vi "Configure.vi"(6 "High Level Config Settings in":T2={"Default Refresh Rate (ms)"=500, "Show Border"=FALSE, "Periodic Decoration Data"=FALSE, "Synchronous Requests"=FALSE, "Reduce Sent Data"=FALSE, "Recommended Control Settings"=FALSE}, 7 "Default Control Behavior":T3, 8 "error in (no error)":errorcluster, 10 "Config Option":T4, 11 "reference in":refnum<class "Web Front Panel.lvclass">) -> (0 "error out":errorcluster, 3 "reference out":refnum<class "Web Front Panel.lvclass">)   [LabVIEW 2017, in "Front Panel Publisher.lvlib" / "Web Front Panel.lvclass"]
doc: "Configure the options for the web-representation of the front panel"
uses:
  Web Front Panel.lvclass
  Controls/FP Object Configuration.ctl
  Common/Enum - Config Option.ctl
  Controls/Cluster - Default Control Behavior.ctl
  Controls/High Level Config Settings.ctl
  Web Front Panel.lvclass/Web Front Panel.ctl
  <vilib>/Utility/error.llb/DialogType.ctl
  Front Panel Objects/Object_class/Object.lvclass
  Front Panel Publisher.lvlib
panel:
  in  "Control Instructions":T1(tab)
  in  "Exit":bool
  in  "Save":bool
  in  "Tab Control":enum32{"Base Config", "Controls", "Indicators"}(tab)
  in  "High Level Config Settings":T2={"Default Refresh Rate (ms)"=750, "Show Border"=FALSE, "Periodic Decoration Data"=FALSE, "Synchronous Requests"=FALSE, "Reduce Sent Data"=FALSE, "Recommended Control Settings"=FALSE}
  in  "Controls":T5[](array[typedef])
  in  "Indicators":T5[](array[typedef])
  # "All controls and indicators can be represented as an image.  Sending a control state as an image means it cannot be interacted with in the web page, and large amounts of data are sent since the whole image is sent instead of just the control value.  This is the Control is Image setting.  This will send just the image but no position or visibility.\n\nThe Image and Visibility will send both the control image, and the position and visibility with each request.  This means if a control is hidden, moved, or resized while the VI is running, the new attributes will be sent automatically.\n\nIf a control is set to Control is Image the position, size, and visibility can be forced to be sent using the Force Update VI.\n\nSince booleans only have two image states, they cannot have the image modes and instead have special Boolean Modes."
  # "When a control is set to Value Only the control's changed position, size or other attributes will not be sent, just the value.  These values will be represented as native web controls and will have the look of the web equivalent control.\n\nThe value is read using get Control Value By Index when possible, but ideally uses no properties or methods on the control.\n\nIf a control is set to Value and Visibility, then value position, size, and other attributes wil be sent with each request.\n\nIf a control is set to Value Only the position, size, and other attributes can be forced to be sent using the Force Update VI."
  # "A Boolean can be set to Value Only, or Value and Visibility like some other controls.  This will have the boolean seen with the web button equivalent.  However since a boolean only has two states there is also the Boolean Value Only which operates like Value Only, except that the two boolean states are seen as images in the webpage, but only send a True or False and not the whole image with each request.\n\nBooleans also have another mode called Boolean Value and Visibility which mirrors the Value and Visibility in that it sends the value, position, size, and other attributes with each request.\n\nIf a control is set to Boolean Value Only the position, size, and other attributes can be forced to be sent using the Force Update VI."
  # "Default Refresh Rate - This is the rate that the page will request new data.  This can be change by clicking the cog in the lower right corner.\n\nShow Border - This will make a border the size of the FP window.\n\nPeriodic Decoration Data - If enabled, then with every request, all decoration positions, size, visibility, and text will be sent and updated.  If false this information will only be updated if a Force Update is used.  Free text is considered a decoration.\n\nSynchronous Requests - This ensures that a request for data won't be sent unless the previous request has been returned.  This is useful at times, but if a reply is lost for some reason the page will hang.\n\nReduce Sent Data - This will reduce the amount of data sent, by only sending data that has changed since the last request from each connection.  This does reduce the amount of data sent, but also increases the time it takes to send a reply."
  # "Control Label"
  # "Control Type"
  # "Display Mode"
  # "Control Label"
  # "Control Type"
  # "Display Mode"
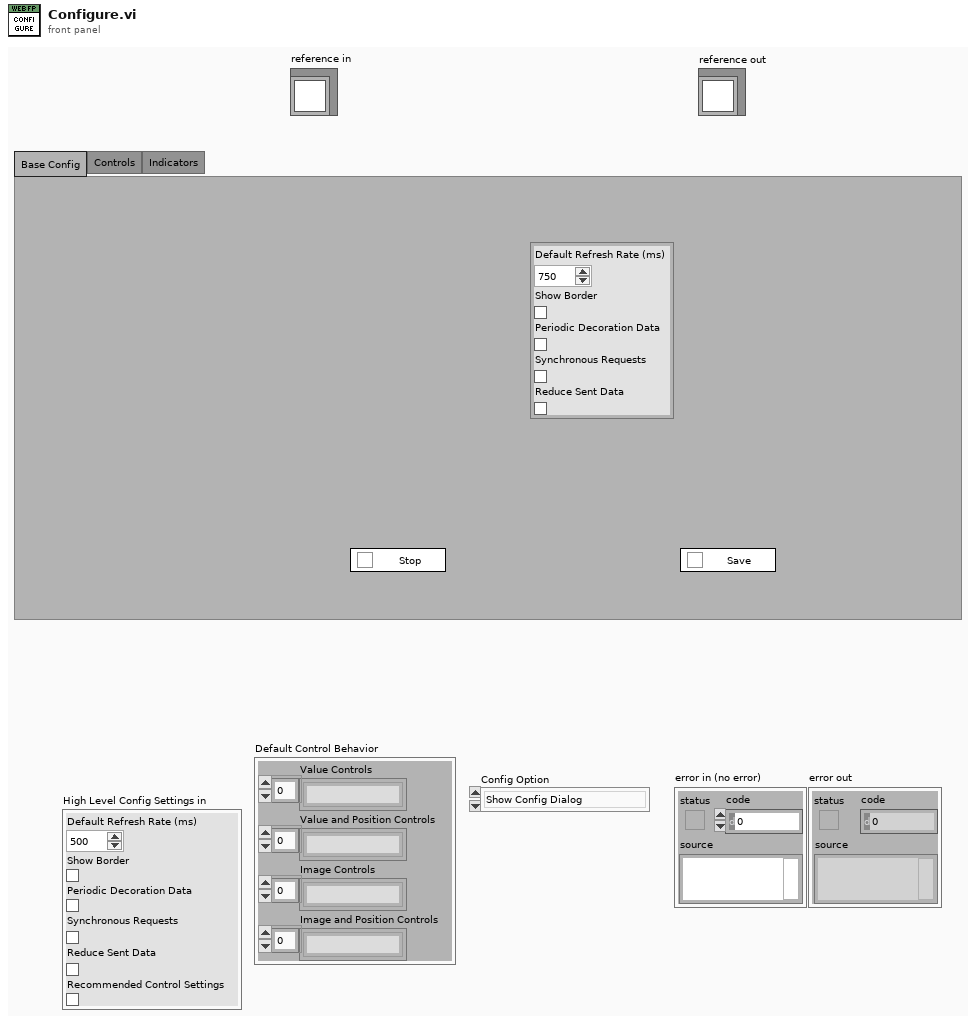
[diagram p1: front panel]
types:
  T1 = enum32{"Image Modes", "Value Modes", "Boolean Modes"}
  T2 = typedef "Front Panel Publisher.lvlib/Web Front Panel.lvclass/High Level Config Settings.ctl" = cluster{"Default Refresh Rate (ms)":i32, "Show Border":bool, "Periodic Decoration Data":bool, "Synchronous Requests":bool, "Reduce Sent Data":bool, "Recommended Control Settings":bool}
  T3 = typedef "Front Panel Publisher.lvlib/Web Front Panel.lvclass/Cluster - Default Control Behavior.ctl" = cluster{"Value Controls":string[], "Value and Position Controls":string[], "Image Controls":string[], "Image and Position Controls":string[]}
  T4 = typedef "Front Panel Publisher.lvlib/Enum - Config Option.ctl" = enum16{"Show Config Dialog", "Don't Show Config Dialog", "Load Config File then Show Dialog", "Load Config File No Dialog"}
  T5 = typedef "Front Panel Publisher.lvlib/Web Front Panel.lvclass/FP Object Configuration.ctl" = cluster{"Name":string, "Control Type":string, "Display Mode":string}
  T6 = enum32{"Invalid", "Standard", "Closed", "Hidden", "Minimized", "Maximized"}
  T7 = typedef "LVPoint32TypeDef.ctl" = cluster{"Horizontal":i32, "Vertical":i32}
  T8 = typedef "Front Panel Publisher.lvlib/Web Front Panel.lvclass/Object Attributes.ctl" = cluster{"VI Identifier":string, "VI Reference":refnum<vi>, "Controls":refnum<class "Object.lvclass">[], "Indicators":refnum<class "Object.lvclass">[], "Decorations":refnum<class "Object.lvclass">[], "VR With Previous Get":refnum<data-value>, "VR With Ring Images":refnum<data-value>}
  T9 = typedef "DialogType.ctl" = u16
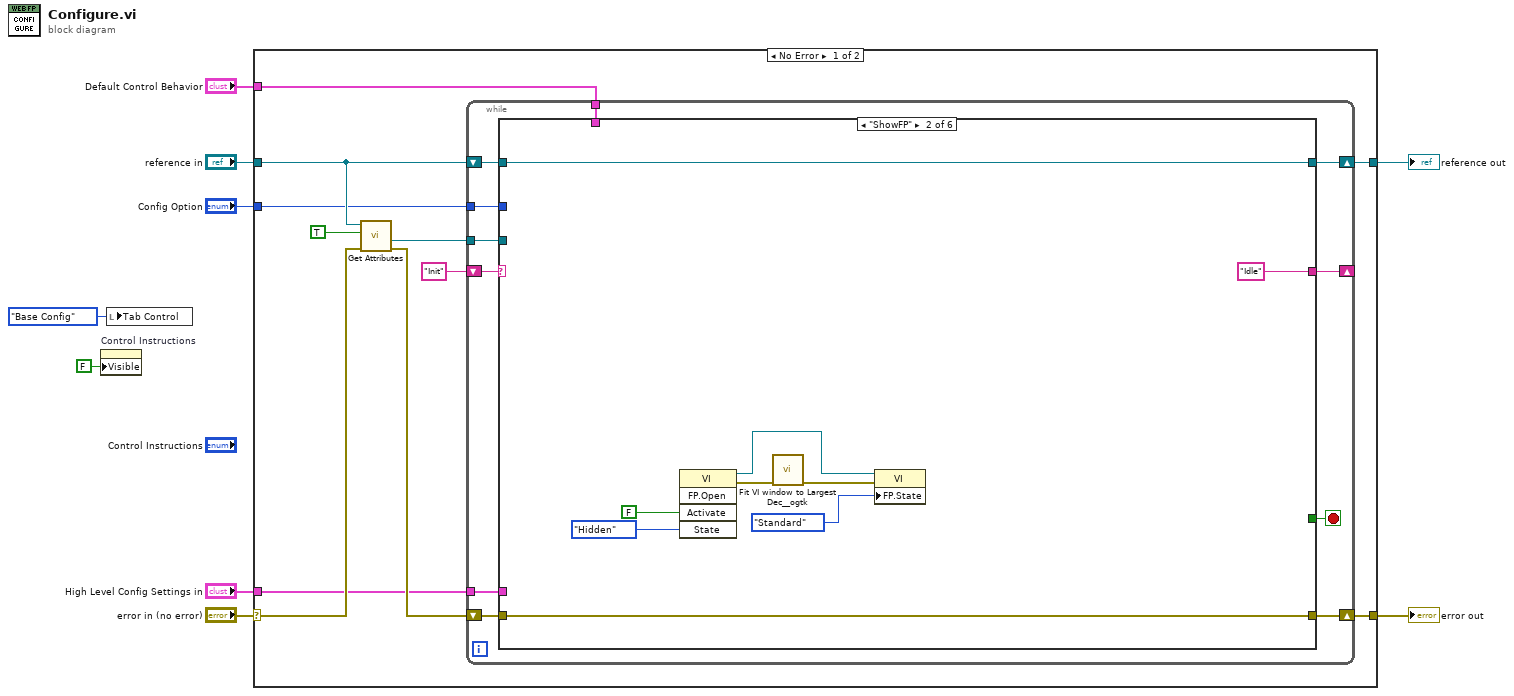
[diagram p0: block diagram]
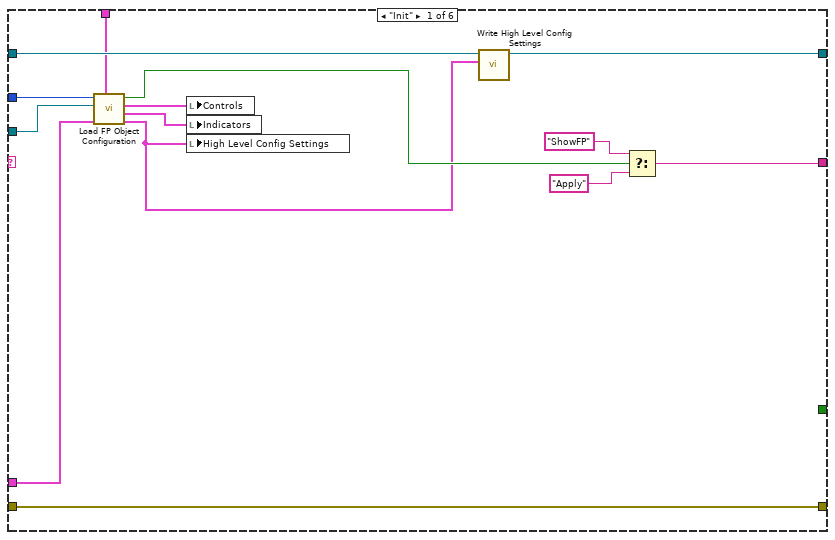
[diagram p2: hidden frame]
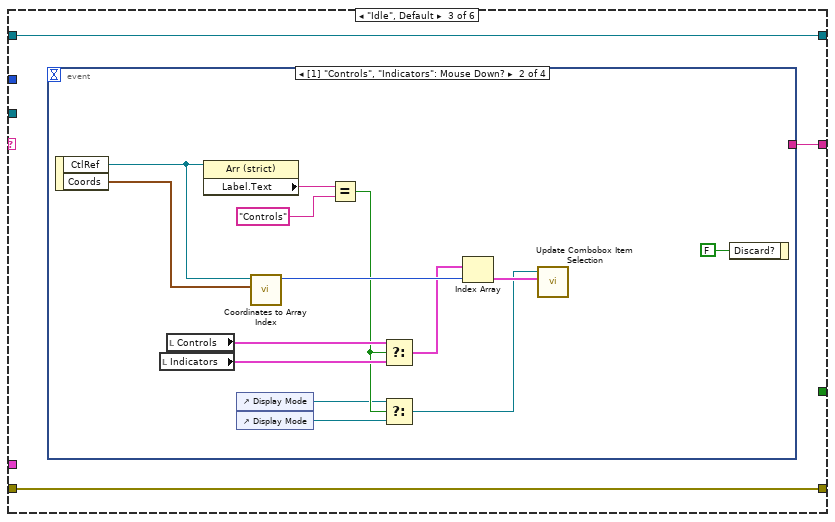
[diagram p3: hidden frame]
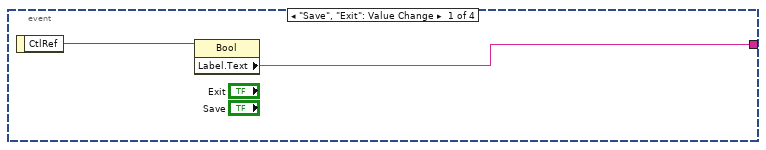
[diagram p4: hidden frame]
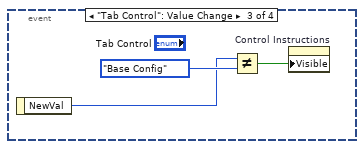
[diagram p5: hidden frame]
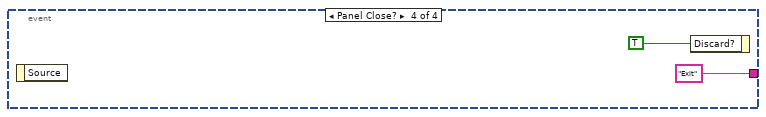
[diagram p6: hidden frame]
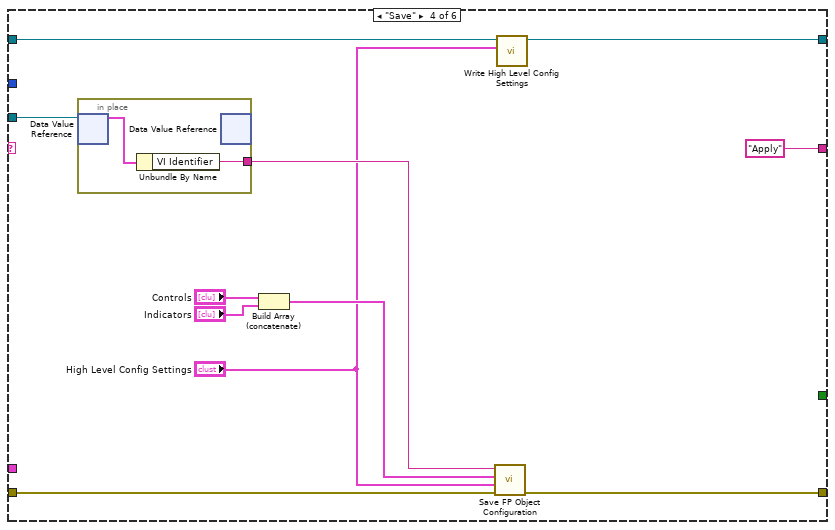
[diagram p7: hidden frame]
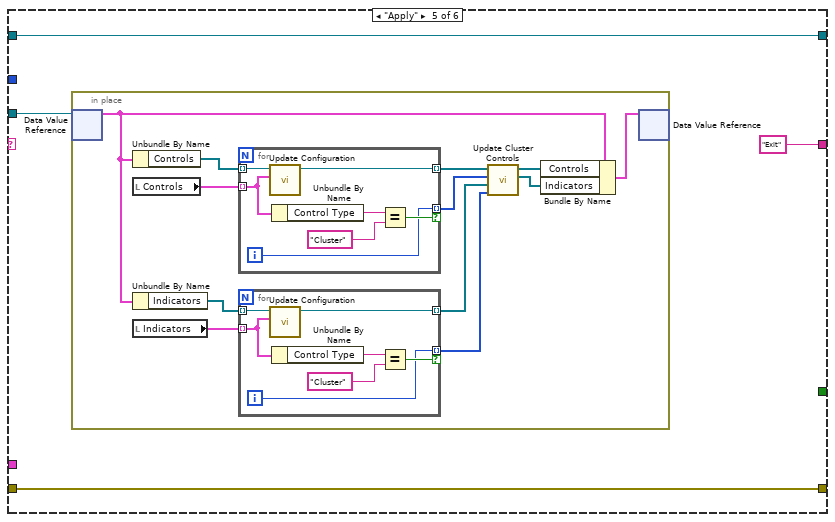
[diagram p8: hidden frame]
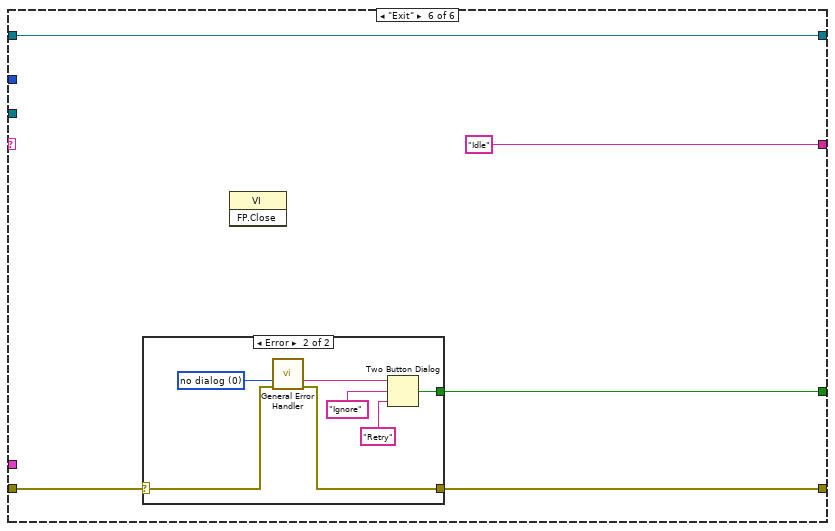
[diagram p9: hidden frame]
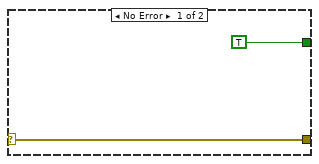
[diagram p10: hidden frame]
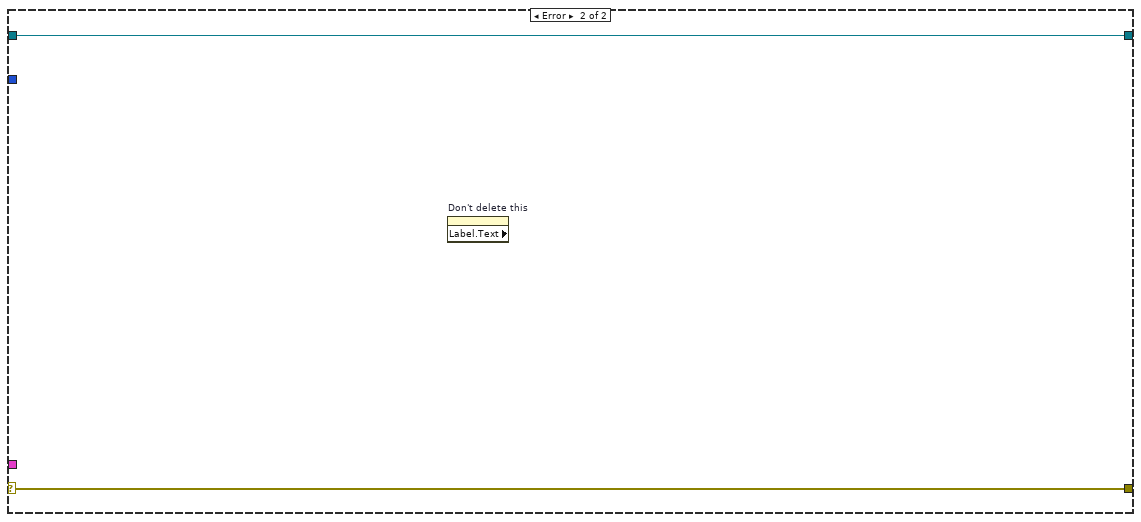
[diagram p11: hidden frame]
diagram:
  n1 = property on="Control Instructions" class="TabCtl (strict)"("Visible"=FALSE) -> ()  [unwired: 2 in, 2 out]
  n2 = local write "Tab Control"(enum32{"Base Config", "Controls", "Indicators"}."Base Config" ("Tab Control")) -> ()
  n3 = case shown="No Error" "error in (no error)" {
    selector: "error in (no error)" -> [w17 w137]
    tunnel: [w20 w137] -> w8
    tunnel: [w12 w136] -> w6
    tunnel: "reference in" -> [w13 w136]
    tunnel: "Default Control Behavior" -> [w14 _]
    tunnel: "High Level Config Settings in" -> [w11 _]
    tunnel: "Config Option" -> [w10 _]
    frame No Error {
      n4 = call "Get Attributes.vi"("error in (no error)"=w17, "Only Get DVR"=TRUE ("OnlyGetDvrReference(False)"), "Web FP In"=w13) -> ("error out"=w16:errorcluster, "DataRef"=w18:refnum<data-value>)  [unwired: 5 in, 2 out]
      n5 = while {
        shift-right: [w30] -> w20
        shift-left: w16 -> [w31]
        shift-right: [w28] -> _
        shift-left: "Init" -> [w29]
        tunnel: w18 -> [w27]
        tunnel: w14 -> [w25]
        shift-right: [w24] -> w12
        shift-left: w13 -> [w23]
        tunnel: w11 -> [w22]
        tunnel: w10 -> [w21]
        stop <- w26 stop-if-true
        n6 = case shown="\"ShowFP\"" w29 {
          tunnel: w31 -> [w45 w54 w56 w86 w93 w125]
          tunnel: [w45 w54 w56 w85 w93 w124] -> w30
          tunnel: [w35 "Idle" w57 "Apply" ("Label.Text") "Exit" ("Label.Text") "Idle" ("Label.Text")] -> w28
          tunnel: w27 -> [w43 _ _ w88 w95 _]
          tunnel: [_ _ _ _ _ w123] -> w26
          tunnel: w25 -> [w41 _ _ _ _ _]
          tunnel: [w33 w47 w55 w80 w92 w122] -> w24
          tunnel: w23 -> [w44 w47 w55 w81 w92 w122]
          tunnel: w22 -> [w40 _ _ _ _ _]
          tunnel: w21 -> [w42 _ _ _ _ _]
          frame "Init" {
            n7 = call "Load FP Object Configuration.vi"("Default Control Behavior"=w41, "High Level Config Settings in"=w40, "DataRef"=w43, "Config Option"=w42) -> ("High Level Config Settings out"=w32:T2, "Indicators"=w39:T5[], "Controls"=w38:T5[], "Show Dialog"=w34:bool)  [unwired: 4 in]
            n8 = local write "Controls"(w38) -> ()
            n9 = local write "Indicators"(w39) -> ()
            n10 = local write "High Level Config Settings"(w32) -> ()
            n11 = call "Write High Level Config Settings.vi"("High Level Config Settings"=w32, "Web FP In"=w44) -> ("Web FP Out"=w33:refnum<class "Web Front Panel.lvclass">)  [unwired: 8 in, 1 out]
            n12 = Select(t="ShowFP", s=w34, f="Apply") -> (s? t:f=w35:string)
          }
          frame "ShowFP" {
            n13 = invoke class="VI" method="FP.Open"("Activate"=FALSE ("Activate?"), "State"=T6."Hidden") -> (reference out=w46:refnum<vi>, error out=w50:errorcluster)  [unwired: 3 in, 3 out]
            n14 = call <userlib>:"Fit VI window to Largest Dec__ogtk.vi"("error in (no error)"=w50) -> ("error out"=w48:errorcluster)  [unwired: 5 in, 1 out]
            n15 = property class="VI"(reference=w46, error in=w48, "FP.State"=T6."Standard" ("Front Panel Window:State")) -> ()  [unwired: 2 out]
          }
          frame "Idle", Default {
            n16 = event shown="[1] \"Controls\", \"Indicators\": Mouse Down?" {
              selector: _ -> [_ _ _ _]
              dyn-events: _ -> [_ _ _ _]
              timeout: _ -> [_ _ _ _]
              tunnel: [w58 _ _ "Exit" ("Label.Text")] -> w57
              event "Save", "Exit": Value Change {
                n17 = event-data() -> ("CtlRef"=w59:refnum<vi>)  [unwired: 1 in]
                n18 = property class="Bool"(reference=w59) -> ("Label.Text"=w58:string)  [unwired: 1 in, 2 out]
              }
              event "Controls", "Indicators": Mouse Down? {
                n19 = event-data() -> ("CtlRef"=w70:refnum<vi>, "Coords"=w69:T7)  [unwired: 1 in]
                n20 = local read "Indicators"() -> (w66:T5[])
                n21 = local read "Controls"() -> (w67:T5[])
                n22 = property class="Arr (strict)"(reference=w70) -> ("Label.Text"=w72:string)  [unwired: 1 in, 2 out]
                n23 = control-ref of="Display Mode"() -> (w63:refnum<vi>)
                n24 = control-ref of="Display Mode"() -> (w62:refnum<vi>)
                n25 = call "Coordinates to Array Index.vi"("Coordinates"=w69, "Array ref"=w70) -> ("Row Index"=w68:i32)  [unwired: 5 in, 4 out]
                n26 = Equal?(x=w72, y="Controls") -> (x = y?=w64:bool)
                n27 = Select(t=w67, s=w64, f=w66) -> (s? t:f=w65:T5[])
                n28 = Select(t=w63, s=w64, f=w62) -> (s? t:f=w60:refnum<vi>)
                n29 = Index Array(array=w65, index=w68) -> (element=w61:T5)
                n30 = call "Update Combobox Item Selection.vi"("Object Config"=w61, "ComboBox in"=w60) -> ()  [unwired: 10 in]
                n31 = event-data("Discard?"=FALSE) -> ()  [unwired: 1 in, 1 out]
              }
              event "Tab Control": Value Change {
                n32 = event-data() -> ("NewVal"=w74:enum32{"Base Config", "Controls", "Indicators"})  [unwired: 1 in]
                n33 = Not Equal?(x=w74, y=enum32{"Base Config", "Controls", "Indicators"}."Base Config") -> (x != y?=w75:bool)
                n34 = property on="Control Instructions" class="TabCtl (strict)"("Visible"=w75) -> ()  [unwired: 2 in, 2 out]
              }
              event Panel Close? {
                n35 = event-data() -> ()  [unwired: 1 in, 1 out]
                n36 = event-data("Discard?"=TRUE) -> ()  [unwired: 1 in, 1 out]
              }
            }
          }
          frame "Save" {
            n37 = in-place {
              in-place-border: [w91] -> w87
              n38 = in-place-dvr #1(w88) -> (w90:T8)  [unwired: 1 out]
              n39 = Unbundle By Name(w90) -> ("VI Identifier"=w91:string)
              n40 = in-place-dvr #1() -> ()  [unwired: 1 in, 2 out]
            }
            n41 = Build Array (concatenate)("Controls", "Indicators") -> (w89:T5[])
            n42 = call "Save FP Object Configuration.vi"("error in (no error)"=w86, "High Level Config Settings"="High Level Config Settings", "Objects Configurations"=w89, "VI Identifier"=w87) -> ("error out"=w85:errorcluster)  [unwired: 7 in]
            n43 = call "Write High Level Config Settings.vi"("High Level Config Settings"="High Level Config Settings", "Web FP In"=w81) -> ("Web FP Out"=w80:refnum<class "Web Front Panel.lvclass">)  [unwired: 8 in, 1 out]
          }
          frame "Apply" {
            n44 = in-place {
              n45 = in-place-dvr #2(w95) -> (w107:T8)  [unwired: 1 out]
              n46 = Unbundle By Name(w107) -> ("Controls"=w106:refnum<class "Object.lvclass">[])
              n47 = local read "Controls"() -> (w105:T5[])
              n48 = Unbundle By Name(w107) -> ("Indicators"=w103:refnum<class "Object.lvclass">[])
              n49 = local read "Indicators"() -> (w102:T5[])
              n50 = for {
                tunnel: w106 -> [w121] mode=indexing
                tunnel: w105 -> [w120] mode=indexing
                tunnel: [w115] -> w101 mode=indexing
                tunnel: [w116] -> w97 mode=indexing if=w117
                i -> [w116]
                n51 = call-dynamic "Update Configuration.vi"("FP Configuration"=w120, "reference in"=w121) -> ("reference out"=w115:refnum<class "Object.lvclass">)  [unwired: 8 in, 1 out]
                n52 = Unbundle By Name(w120) -> ("Control Type"=w119:string)
                n53 = Equal?(x=w119, y="Cluster") -> (x = y?=w117:bool)
              }
              n54 = for {
                tunnel: w103 -> [w114] mode=indexing
                tunnel: w102 -> [w113] mode=indexing
                tunnel: [w110] -> w99 mode=indexing
                tunnel: [w108] -> w96 mode=indexing if=w109
                i -> [w108]
                n55 = call-dynamic "Update Configuration.vi"("FP Configuration"=w113, "reference in"=w114) -> ("reference out"=w110:refnum<class "Object.lvclass">)  [unwired: 8 in, 1 out]
                n56 = Unbundle By Name(w113) -> ("Control Type"=w112:string)
                n57 = Equal?(x=w112, y="Cluster") -> (x = y?=w109:bool)
              }
              n58 = call "Update Cluster Controls.vi"("Cluster Indicator Indexes"=w96, "Indicators In"=w99, "Cluster Control Indexes"=w97, "Controls In"=w101) -> ("Indicators Out"=w98:refnum<class "Object.lvclass">[], "Controls Out"=w100:refnum<class "Object.lvclass">[])  [unwired: 6 in]
              n59 = Bundle By Name(cluster=w107, "Controls"=w100, "Indicators"=w98) -> (w104:T8)
              n60 = in-place-dvr #2(w104) -> ()  [unwired: 2 out]
            }
          }
          frame "Exit" {
            n61 = case shown="Error" w125 {
              selector: w125 -> [w128 w135]
              tunnel: [w128 w134] -> w124
              tunnel: [TRUE ("T button?") w129] -> w123
              frame No Error {
              }
              frame Error {
                w133 = T9 0 items=["no dialog", "OK message", "continue or stop message", "OK message + warnings", "continue/stop + warnings"] ("type of dialog (OK msg:1)")
                n62 = call <vilib>:"General Error Handler.vi"("type of dialog (OK msg:1)"=w133, "error in (no error)"=w135) -> ("message"=w132:string, "error out"=w134:errorcluster)  [unwired: 9 in, 3 out]
                n63 = Two Button Dialog(message=w132, 1:"Retry", 2:"Ignore" ("String")) -> (T button?=w129:bool)
              }
            }
            n64 = invoke class="VI" method="FP.Close"() -> ()  [unwired: 3 in, 3 out]
          }
        }
      }
    }
    frame Error {
      n65 = property on="Don't delete this" class="LVClassControl (strict)" props=["Label", "Text"]() -> ()  [unwired: 2 in, 3 out]
    }
  }
  "error out" <- w8
  "reference out" <- w6
